vi "arrayWaveform.vi"() -> ()   [LabVIEW 2021]
panel:
  out "Waveform Graph":dbl[][](graph)
  in  "My Array":dbl[][](array[numeric])
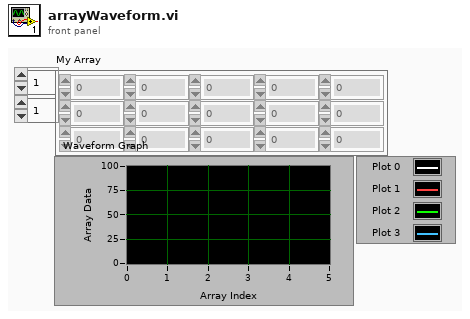
[diagram p1: front panel]
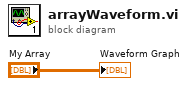
[diagram p0: block diagram]
diagram:
  "Waveform Graph" <- "My Array"
